vi "Set Variant Property.vi"(6 "Control Ref Queue":T1, 8 "error in (no error)":errorcluster, 10 "Property In":variant, 11 "3D Comet.lvclass in":refnum<class "3D Comet.lvclass">) -> (0 "error out":errorcluster, 3 "3D Comet.lvclass":refnum<class "3D Comet.lvclass">)   [LabVIEW 2020, in "3D Comet.lvclass"]
uses:
  <vilib>/Math Plots/3D Math Plots/3D Comet/3D Comet/3D Comet.lvclass
  <vilib>/Math Plots/3D Math Plots/3D Comet/3D Comet/Typedef/3D Comet Property Array.ctl
  <vilib>/Math Plots/3D Math Plots/3D Comet/3D Comet/Typedef/3D Comet Property.ctl
  <vilib>/Math Plots/3D Math Plots/3D Plot/3D Plot/Typedef/Sprite Type.ctl
  <vilib>/Math Plots/3D Math Plots/3D Plot/3D Plot/Typedef/Line Type.ctl
  <vilib>/Math Plots/3D Math Plots/3D Plot/Action String/3DMathPlot Ctrl Act Queue.ctl
  <vilib>/Math Plots/3D Math Plots/3D Plot/Action String/3DMathPlot Ctrl Act Cluster.ctl
  <vilib>/Math Plots/3D Math Plots/3D Plot/Action String/3DMathPlot State Class.ctl
  <vilib>/Math Plots/3D Math Plots/3D Comet/3D Comet/3D Comet.lvclass/3D Comet.ctl
  <vilib>/Math Plots/3D Math Plots/3D Plot/3D Plot/3D Plot.lvclass
panel:
  in  "3D Comet Property Array":T2
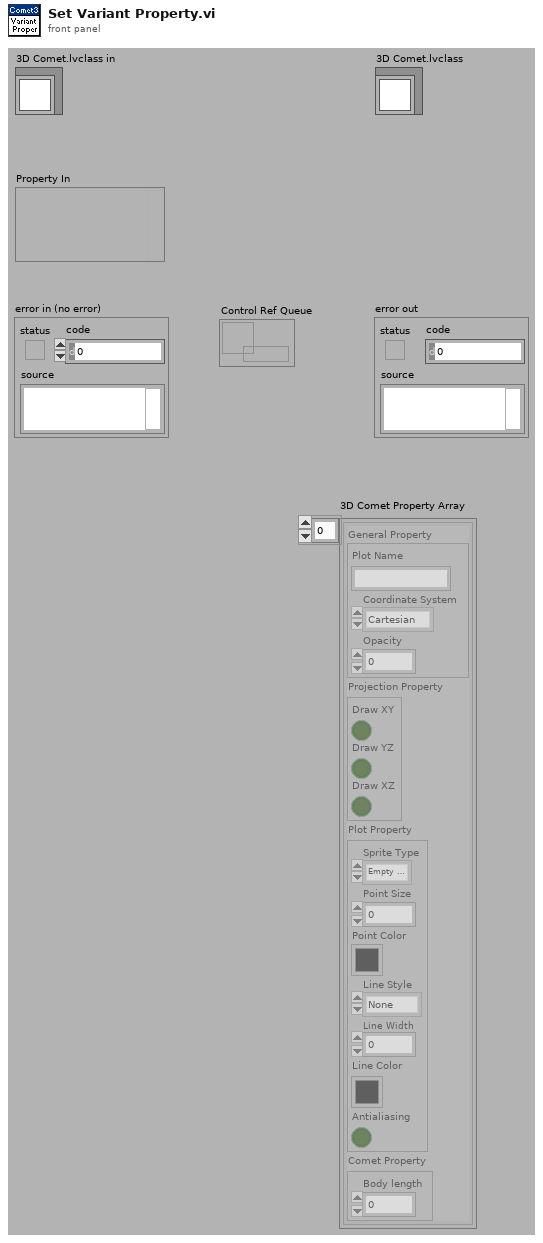
[diagram p1: front panel]
types:
  T1 = typedef "3DMathPlot Ctrl Act Queue.ctl" = refnum<queue>
  T2 = typedef "3D Comet.lvclass/3D Comet Property Array.ctl" = T3[]
  T3 = typedef "3D Comet.lvclass/3D Comet Property.ctl" = cluster{"General Property":cluster{"Plot Name":string, "Coordinate System":enum16{"Cartesian", "Cylindrical", "Spherical"}, "Opacity":sgl}, "Projection Property":cluster{"Draw XY":bool, "Draw YZ":bool, "Draw XZ":bool}, "Plot Property":cluster{"Sprite Type":T4, "Point Size":sgl, "Point Color":u32, "Line Style":T5, "Line Width":sgl, "Line Color":u32, "Antialiasing":bool}, "Comet Property":cluster{"Body length":sgl}}
  T4 = typedef "3D Plot.lvclass/Sprite Type.ctl" = enum16{"None", "Empty Square", "Solid Square", "Empty Diamond", "Solid Diamond", "Empty Circle", "Solid Circle", "Asterisk", "Bold X", "Wireframe Sphere", "Solid Sphere", "Wireframe Cube", "Solid Cube"}
  T5 = typedef "3D Plot.lvclass/Line Type.ctl" = enum16{"None", "Solid", "Dash", "Dot", "Dash Dot"}
  T6 = typedef "3DMathPlot State Class.ctl" = enum16{"Update All Objects (Undo)", "Update Light Object Only", "Update Axis Object Only", "Update Plot Object Only", "Update Cursor Object Only", "Update Axis Plot Cursor Objects", "No Update"}
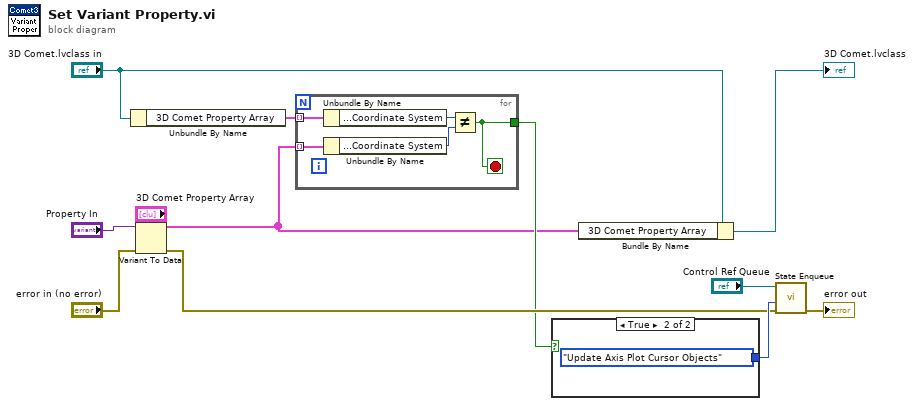
[diagram p0: block diagram]
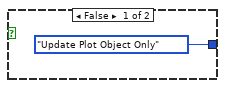
[diagram p2: hidden frame]
diagram:
  n1 = Unbundle By Name("3D Comet.lvclass in") -> ("3D Comet Property Array"=w8:T2)
  n2 = Variant To Data(error in="error in (no error)", type="3D Comet Property Array", Variant="Property In") -> (data=w2:T2, error out=w5:errorcluster)
  n3 = for {
    tunnel: w2 -> [w16] mode=indexing
    tunnel: w8 -> [w17] mode=indexing
    tunnel: [w13] -> w3
    stop <- w13 stop-if-true
    n4 = Unbundle By Name(w17) -> ("General Property.Coordinate System"=w15:enum16{"Cartesian", "Cylindrical", "Spherical"})
    n5 = Unbundle By Name(w16) -> ("General Property.Coordinate System"=w14:enum16{"Cartesian", "Cylindrical", "Spherical"})
    n6 = Not Equal?(x=w15, y=w14) -> (x != y?=w13:bool)
  }
  n7 = case shown="True" w3 {
    tunnel: [3DMathPlot_State_Class."Update Plot Object Only" ("Display State Change Class") 3DMathPlot_State_Class."Update Axis Plot Cursor Objects" ("Display State Change Class")] -> w7
    frame False {
    }
    frame True {
    }
  }
  n8 = Bundle By Name(cluster="3D Comet.lvclass in", "3D Comet Property Array"=w2) -> (→"3D Comet.lvclass":refnum<class "3D Comet.lvclass">)
  n9 = call <vilib>:"State Enqueue.vi"("error in (no error)"=w5, "Display State Change Class"=w7, "Control Ref Queue"="Control Ref Queue") -> ("error out"=→"error out":errorcluster)  [unwired: 8 out]
